vi "NI VeriStand - Get Fault List.vi"(8 "error in (no error)":errorcluster, 11 "ChannelFault in":T1) -> (0 "error out":errorcluster, 1 "Values":dbl[](array[numeric]), 2 "Channels":string[](array[string]), 3 "ChannelFault out":T1)   [LabVIEW 2020, in "NI_VS ChannelFault ExecutionAPI.lvlib"]
doc: "Returns a list of all faulted channels. You can create faulted channels manually using the Channel Fault Manager tool or programmatically using the Set Fault Value VI."
uses:
  <vilib>/NI VeriStand/Execution/ChannelFaultManager/NI_VS ChannelFault ExecutionAPI.lvlib
  <vilib>/NI VeriStand/Execution/ChannelFaultManager/ChannelFaultAPI.ctl
  NationalInstruments.VeriStand.ClientAPI
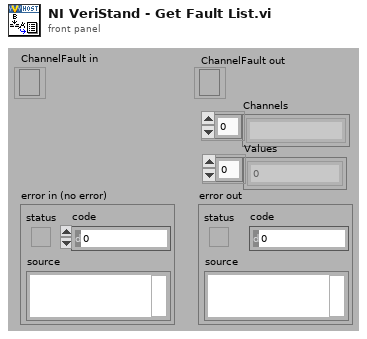
[diagram p1: front panel]
types:
  T1 = typedef "NI_VS ChannelFault ExecutionAPI.lvlib/ChannelFaultAPI.ctl" = refnum<k24>
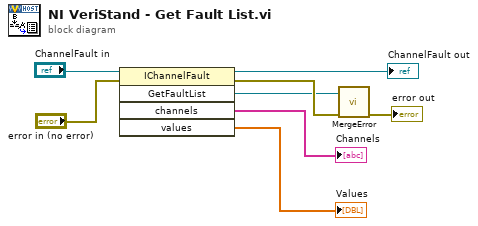
[diagram p0: block diagram]
diagram:
  n1 = invoke class="IChannelFault" method="GetFaultList"(reference="ChannelFault in", error in="error in (no error)") -> (reference out=→"ChannelFault out":T1, error out=w6:errorcluster, "GetFaultList"=w5:refnum<k24>, "channels"=→"Channels":string[], "values"=→"Values":dbl[])  [unwired: 3 in]
  n2 = call <vilib>:"MergeError.vi"("error in (no error)"=w6, "Error"=w5) -> ("error out"=→"error out":errorcluster)  [unwired: 9 out]
